vi "XML Get Acquisition Chassis.vi"(11 "Acquisition Network":T2) -> (1 "Acquisition Chassis Names":string[](array[string]), 2 "Number of BPM Readings":i32, 3 "Acquisition Variable Names":string[][](array[string]), 4 "Inverse BPM Matrix Mapping":u32[][](array[numeric]), 5 "BPM Parameters":T1[](array[typedef]), 6 "BPM Matrix Mapping":cluster{u32[]}[](array[cluster]), 7 "Selected BPM Readings":u32[](array[numeric]))   [LabVIEW 2011, in "XML VIs.lvlib"]
doc: "Extracts the Acquisition Network configuration data (ordered by chassis-by-chassis) and builds dedicated clusters for each configuration (ordered by response matrix row indexes)."
uses:
  XML VIs.lvlib
  Types Definitions/Type Acquisition Network Configuration.ctl
  Types Definitions/Type BPM Parameters.ctl
  Type Definitions.lvlib
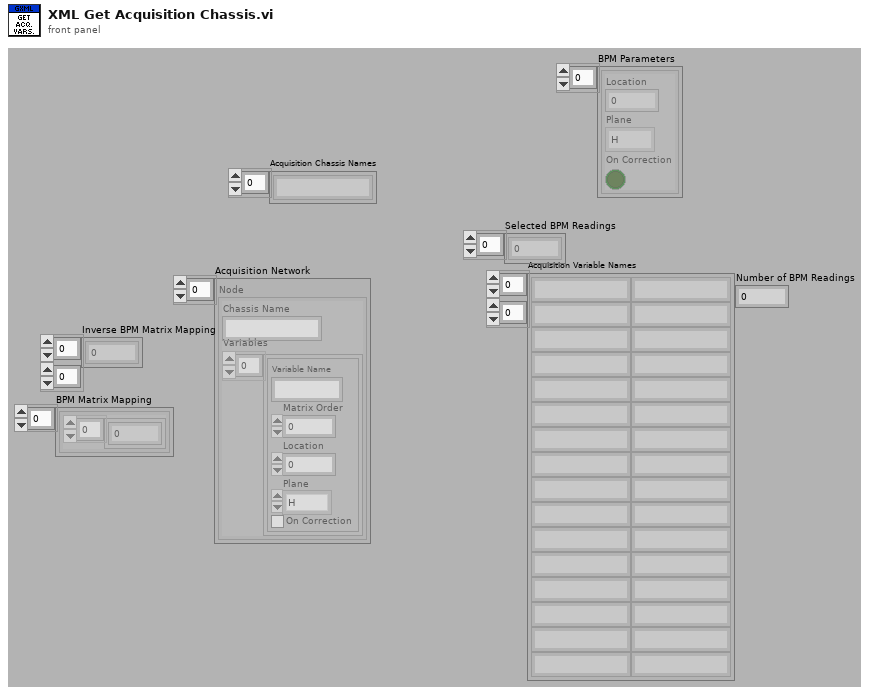
[diagram p1: front panel]
types:
  T1 = typedef "Type Definitions.lvlib/Type BPM Parameters.ctl" = cluster{"Location":dbl, "Plane":enum8{"H", "V"}, "On Correction":bool}
  T2 = typedef "Type Definitions.lvlib/Type Acquisition Network Configuration.ctl" = cluster{"Chassis Name":string, "Variables":cluster{"Variable Name":string, "Matrix Order":u32, "Location":dbl, "Plane":enum8{"H", "V"}, "On Correction":bool}[]}[]
  T3 = cluster{"Variable Name":string, "Matrix Order":u32, "Location":dbl, "Plane":enum8{"H", "V"}, "On Correction":bool}[]
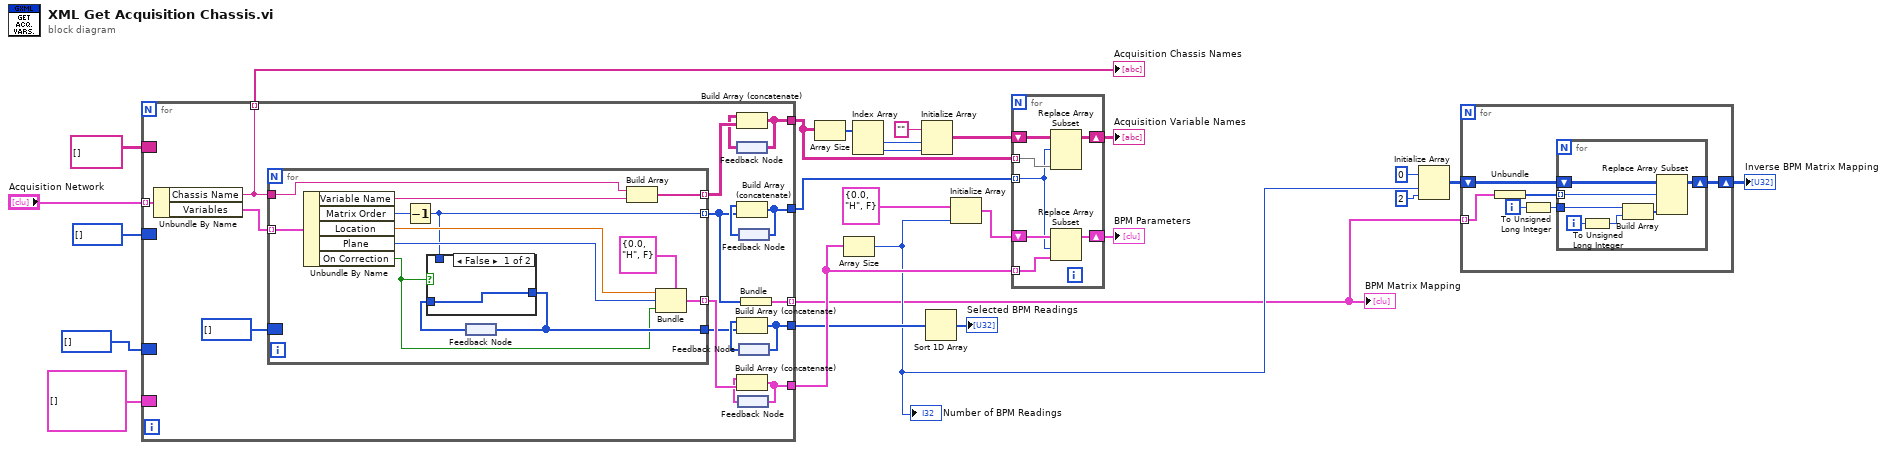
[diagram p0: block diagram]
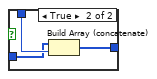
[diagram p2: hidden frame]
diagram:
  n1 = for {
    tunnel: "Acquisition Network" -> [w43] mode=indexing
    tunnel: [w39] -> w18 mode=indexing
    tunnel: [w30] -> w8
    tunnel: [w36] -> w13
    border: T1[] [] -> [_]
    border: u32[] [] -> [_]
    border: string[][] [] -> [_]
    tunnel: [w33] -> w11
    tunnel: [w32] -> w10
    border: u32[] [] -> [_]
    tunnel: [w27] -> w1 mode=indexing
    n2 = Unbundle By Name(w43) -> ("Chassis Name"=w39:string, "Variables"=w42:T3)
    n3 = for {
      tunnel: w42 -> [w56] mode=indexing
      tunnel: w39 -> [w54]
      tunnel: [w47] -> w28 mode=indexing
      tunnel: [w53] -> w41 mode=indexing
      tunnel: [w48] -> w38 mode=indexing
      tunnel: [w45] -> w29
      border: u32[] [] -> [_]
      n4 = Unbundle By Name(w56) -> ("Variable Name"=w55:string, "Matrix Order"=w52:u32, "Location"=w51:dbl, "Plane"=w50:enum8{"H", "V"}, "On Correction"=w44:bool)
      n5 = Decrement(x=w52) -> (x-1=w47:u32)
      n6 = feedback #1() -> (w46:u32[])
      n7 = case shown="False" w44 {
        tunnel: w47 -> [_ w60]
        tunnel: w46 -> [w57 w59]
        tunnel: [w57 w58] -> w45
        frame False {
        }
        frame True {
          n8 = Build Array (concatenate)(w59, w60) -> (w58:u32[])
        }
      }
      n9 = feedback-in #1(w45) -> ()
      n10 = Build Array(w54, w55) -> (w53:string[])
      n11 = Bundle(cluster=T1 {"Location"=0.0, "Plane"=enum."H", "On Correction"=FALSE} ("BPM Parameters"), "Location"=w51, "Plane"=w50, "On Correction"=w44) -> (w48:T1)
    }
    n12 = feedback #2() -> (w40:string[][])
    n13 = Build Array (concatenate)(w40, w41) -> (w33:string[][])
    n14 = feedback-in #2(w33) -> ()
    n15 = feedback #3() -> (w37:T1[])
    n16 = Build Array (concatenate)(w37, w38) -> (w36:T1[])
    n17 = feedback-in #3(w36) -> ()
    n18 = feedback #4() -> (w34:u32[])
    n19 = Build Array (concatenate)(w34, w28) -> (w32:u32[])
    n20 = feedback-in #4(w32) -> ()
    n21 = feedback #5() -> (w31:u32[])
    n22 = Build Array (concatenate)(w31, w29) -> (w30:u32[])
    n23 = feedback-in #5(w30) -> ()
    n24 = Bundle(w28) -> (w27:cluster{u32[]})  [unwired: 1 in]
  }
  "Acquisition Chassis Names" <- w18
  "BPM Matrix Mapping" <- w1
  n25 = Array Size(array=w11) -> (size(s)=w26:i32[])
  n26 = Array Size(array=w13) -> (size(s)=w2:i32)
  "Number of BPM Readings" <- w2
  n27 = Index Array(array=w26) -> (element #1=w25:i32, element #2=w24:i32)  [unwired: 2 in]
  n28 = Initialize Array("" ("element"), w25, w24) -> (w23:string[][])
  n29 = Sort 1D Array(array=w8) -> (sorted array=→"Selected BPM Readings":u32[])
  n30 = Initialize Array(T1 {"Location"=0.0, "Plane"=enum."H", "On Correction"=FALSE} ("BPM Parameters"), w2) -> (w15:T1[])
  n31 = for {
    shift-right: [w66] -> w21
    shift-left: w23 -> [w67]
    tunnel: w11 -> [w65] mode=indexing
    tunnel: w10 -> [w61] mode=indexing
    shift-right: [w63] -> w14
    shift-left: w15 -> [w64]
    tunnel: w13 -> [w62] mode=indexing
    n32 = Replace Array Subset(array=w67, new element=w65, index (row)=w61) -> (w66:string[][])  [unwired: 1 in]
    n33 = Replace Array Subset(array=w64, new element=w62, index=w61) -> (w63:T1[])
  }
  "Acquisition Variable Names" <- w21
  "BPM Parameters" <- w14
  n34 = Initialize Array(u32 0 ("element"), w2, 2 ("dimension size")) -> (w4:u32[][])
  n35 = for {
    shift-right: [w72] -> w3
    shift-left: w4 -> [w73]
    tunnel: w1 -> [w69] mode=indexing
    i -> [w71]
    n36 = Unbundle(w69) -> (w68:u32[])
    n37 = To Unsigned Long Integer(number=w71) -> (unsigned 32bit integer=w70:u32)
    n38 = for {
      tunnel: w70 -> [w78]
      shift-right: [w79] -> w72
      shift-left: w73 -> [w80]
      tunnel: w68 -> [w76] mode=indexing
      i -> [w74]
      n39 = To Unsigned Long Integer(number=w74) -> (unsigned 32bit integer=w75:u32)
      n40 = Build Array(w78, w75) -> (w77:u32[])
      n41 = Replace Array Subset(array=w80, new element=w77, index (row)=w76) -> (w79:u32[][])  [unwired: 1 in]
    }
  }
  "Inverse BPM Matrix Mapping" <- w3
